vi "Main.vi"   [LabVIEW 2021]
uses:
  APG/APG/APG.lvclass
  C:/Program Files/National Instruments/LabVIEW 2021/vi.lib/ActorFramework/Actor/Actor.lvclass
  <vilib>/ActorFramework/Actor/Actor.lvclass
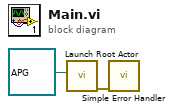
[diagram p0: block diagram]
diagram:
  n1 = call <vilib>:"Launch Root Actor.vi"("Actor"=refnum<class "APG.lvclass"> refnum ("APG.lvlib:APG.lvclass")) -> ("error out"=w1:errorcluster)  [unwired: 9 in, 1 out]
  n2 = call <vilib>:"Simple Error Handler.vi"("error in (no error)"=w1) -> ()  [unwired: 4 in, 5 out]
